vi "Write Simulator.lvclass 1.vi"(8 "error in (no error)":errorcluster, 10 "Simulator.lvclass":refnum<class "Simulator.lvclass">, 11 "Measurement2D in":refnum<class "Measurement2D.lvclass">) -> (0 "error out":errorcluster, 3 "Measurement2D out":refnum<class "Measurement2D.lvclass">)   [LabVIEW 2018, in "Measurement2D.lvclass"]
uses:
  Measurement2D.lvclass
  Instrument/Simulator/Simulator.lvclass
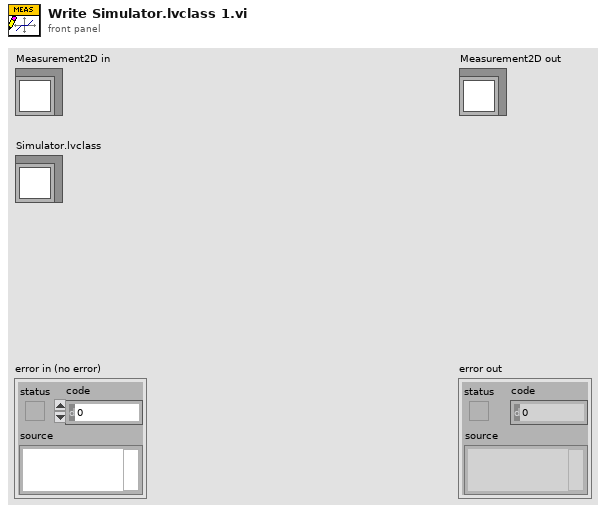
[diagram p1: front panel]
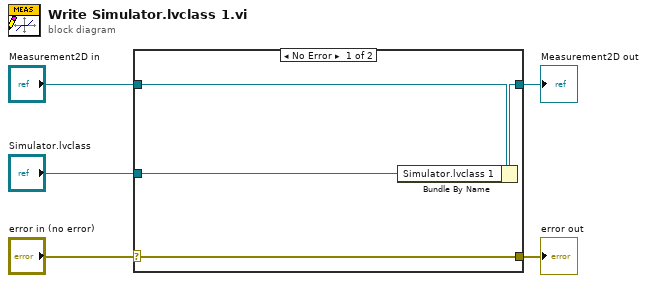
[diagram p0: block diagram]
diagram:
  n1 = case shown="No Error" "error in (no error)" {
    selector: "error in (no error)" -> [w9 w10]
    tunnel: [w9 w10] -> w4
    tunnel: [w7 w11] -> w2
    tunnel: "Measurement2D in" -> [w8 w11]
    tunnel: "Simulator.lvclass" -> [w6 _]
    frame No Error {
      n2 = Bundle By Name(cluster=w8, "Simulator.lvclass 1"=w6) -> (w7:refnum<class "Measurement2D.lvclass">)
    }
    frame Error {
    }
  }
  "error out" <- w4
  "Measurement2D out" <- w2
